vi "SetHSSpeedSD.vi"(3 "error in (no error)":errorcluster, 4 "index":i32, 5 "type":T1) -> (0 "error out":errorcluster, 1 "DLL error code":u32)   [LabVIEW 2015]
doc: "This function will set the horizontal speed to one of the possible speeds of the system. It will be used for subsequent acquisitions.\n\n<B>Parameters:</B>\ntype - the horizontal read mode.\n Valid values: 0 - speed of data readout.\n 1 - speed of binning.\n 2 - speed of dumping pixels.\nindex - the horizontal speed to be used\n Valid values: 0 to <B>GetNumberHSSpeeds</B>-1\n\n<B>Error codes:</B>\nDRV_SUCCESS - Horizontal speed set.\nDRV_NOT_INITIALIZED - System not initialized.\nDRV_ACQUIRING - Acquisition in progress.\nDRV_P1INVALID - Mode is invalid.\nDRV_P2INVALID - Index is out off range."
uses:
  atmcd32d.llb/HSSpeed_type typedef.ctl
  DLL/atmcd32d.dll
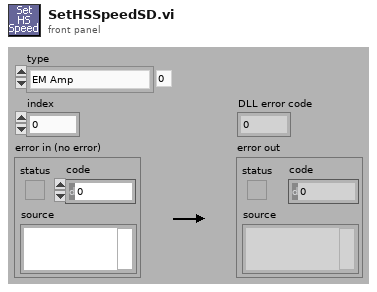
[diagram p1: front panel]
types:
  T1 = typedef "HSSpeed_type typedef.ctl" = enum16{"EM Amp", "Conventional Amp"}
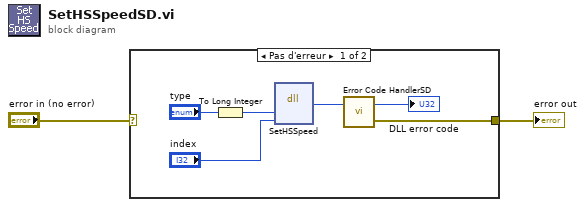
[diagram p0: block diagram]
diagram:
  n1 = case shown="Pas d'erreur" "error in (no error)" {
    selector: "error in (no error)" -> [_ w9]
    tunnel: [w7 w9] -> w1
    frame No Error {
      n2 = To Long Integer(number="type") -> (32bit integer=w4:i32)
      n3 = dll-call lib="G:/SD/TRANCON/DLL/Atmcd32d.dll" fn="SetHSSpeed"("type"=w4, "index"="index") -> (w8:u32)  [unwired: 5 in, 2 out]
      n4 = call "Error Code HandlerSD.vi"("DLL error code"=w8) -> ("error out"=w7:errorcluster, "dup DLL error code"=→"DLL error code":u32)  [unwired: 1 in]
    }
    frame Error {
    }
  }
  "error out" <- w1
